vi "bigcryo_Harry-IcH - v5.vi"() -> ()   [LabVIEW 2019]
uses:
  Global 2.vi
  <vilib>/Utility/file.llb/Read From Spreadsheet File (DBL).vi
panel:
  out "Sample Temp [K] - Meas":dbl=1.55928
  out "Sample Temp - Idle [K]":dbl
  in  "LakeShore340":refnum<visa-resource-name>="COM7"
  out "dV/dI-I":cluster{dbl[], dbl[]}(graph) caption="XY Graph"
  out "I-V":cluster{dbl[], dbl[]}(graph) caption="XY Graph"
  out "Status":string="Welcome!"
  in  "Stop":bool
  in  "Keithley":refnum<visa-resource-name>="GPIB1::20::INSTR"
  in  "Delay [sec]":dbl=0.002 format="%#_6e"
  in  "Compliance [V] 2":dbl=10.0 format="%#_6f"
  in  "Delta [A]":dbl=1e-05 format="%#_6e"
  in  "Abort Conductance":bool
  in  "Step [A]":dbl=1e-05 format="%#_6e"
  in  "I-Max [A]":dbl=0.002 format="%#_6e"
  in  "Arm Conductance":bool
  in  "Measure":bool
  in  "Directory Output":string="C:\\User Data\\hlb54\\210111_42B\\JJ1\\IcH_pos_to_neg_T=4p00K_set=0p0T"
  out "B Now":string="-0.202"
  out "error out 6":errorcluster
  in  "Minicryo":bool=TRUE
  in  "Field and rate":dbl[][](array[numeric])
  in  "step":bool=TRUE
  in  "Set Rate (T/min)":dbl=0.1
  in  "Magnet VISA?":refnum<visa-resource-name>="COM6"
  out "?":refnum<visa-resource-name>="GPIB0::20::INSTR"
  out "Iteration?":i32=401
  out "Path Out":path=path "C:/User Data/Sachio/gigi.dat"
  in  "Start Field (T)":dbl=0.2 format="%#_7f"
  in  "Mag Field Step":dbl=0.002
  out "B Aim":dbl=-0.202
  in  "Stop Field":dbl=-0.2
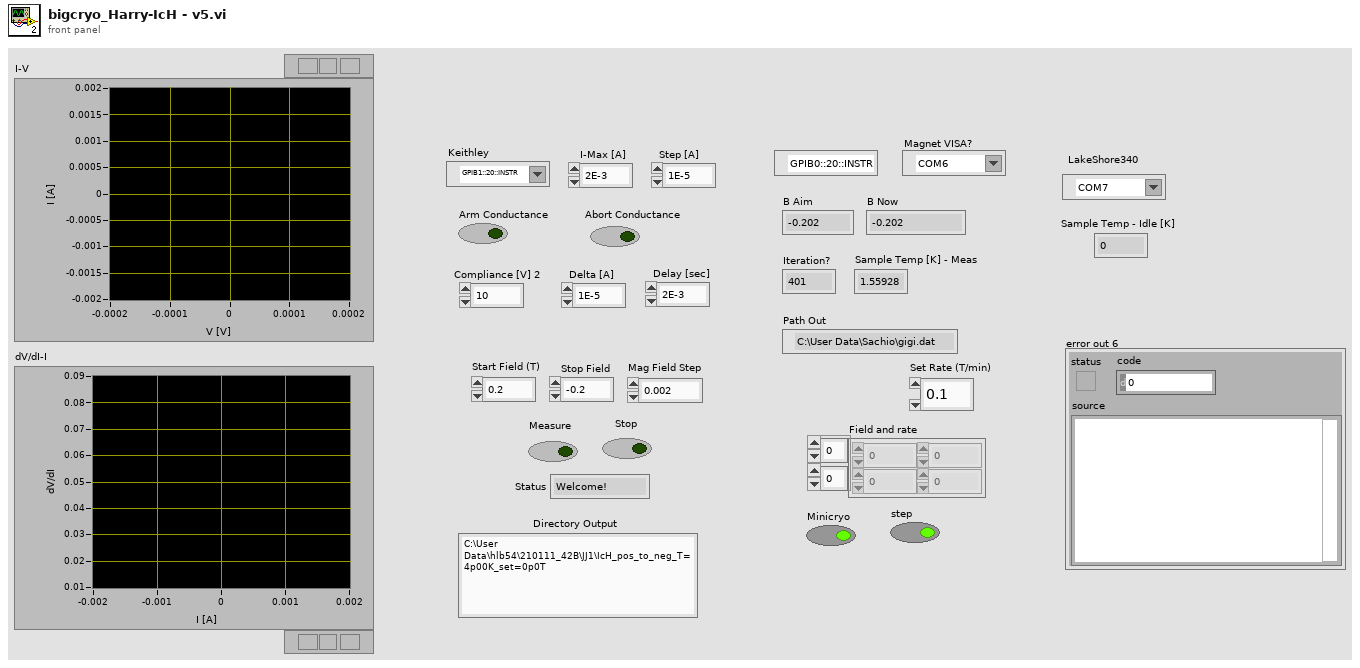
[diagram p1: front panel]
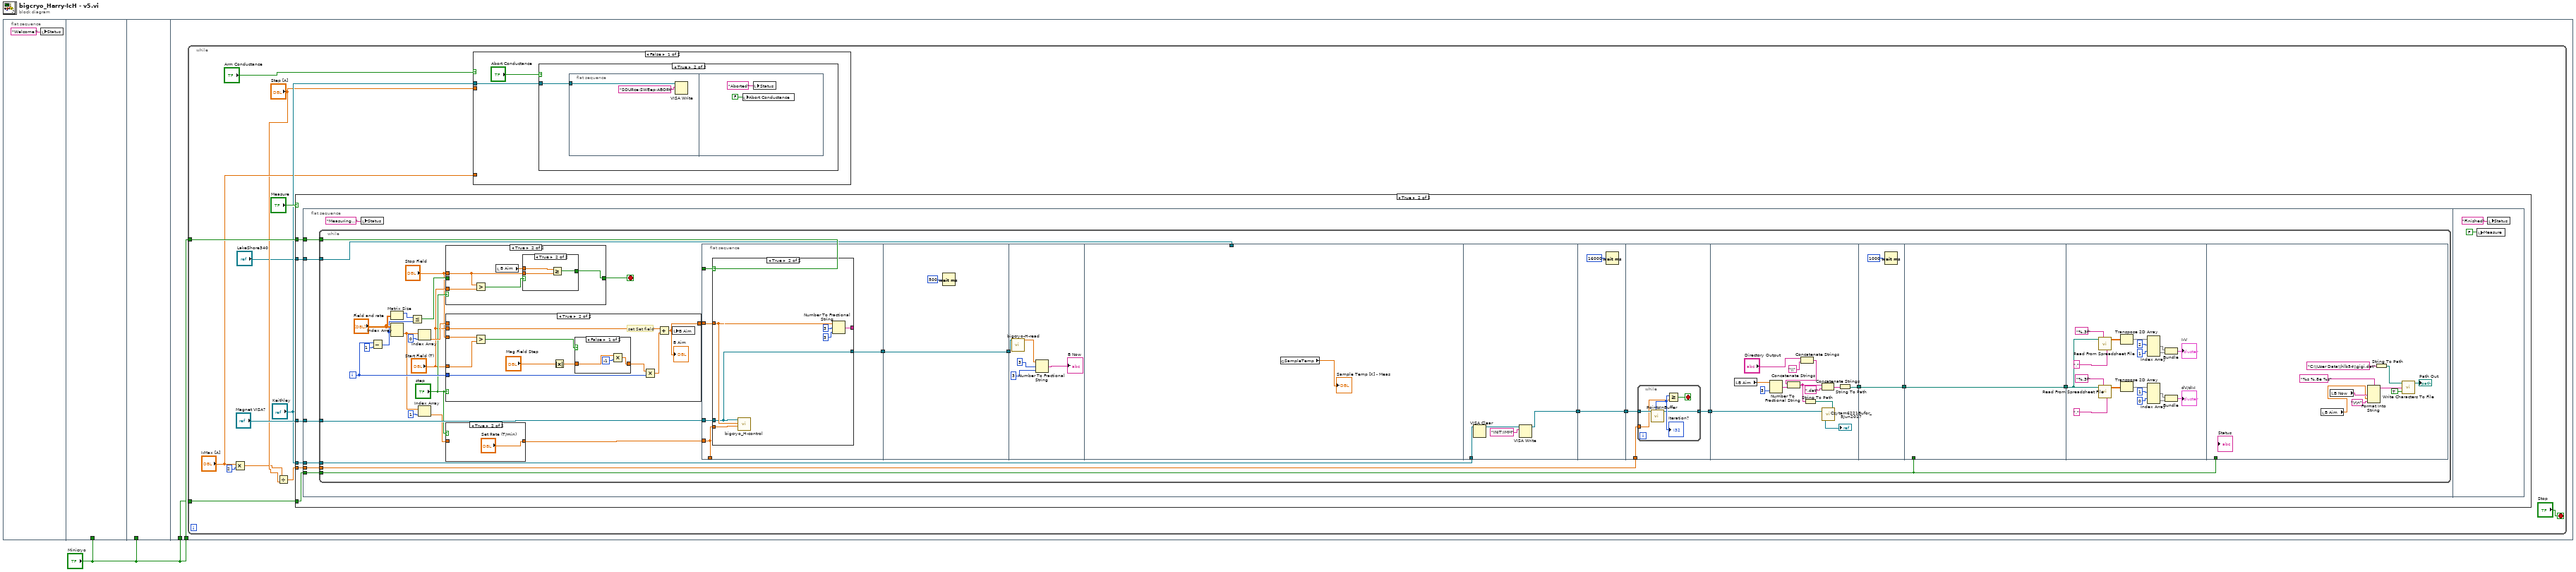
[diagram p0: block diagram]
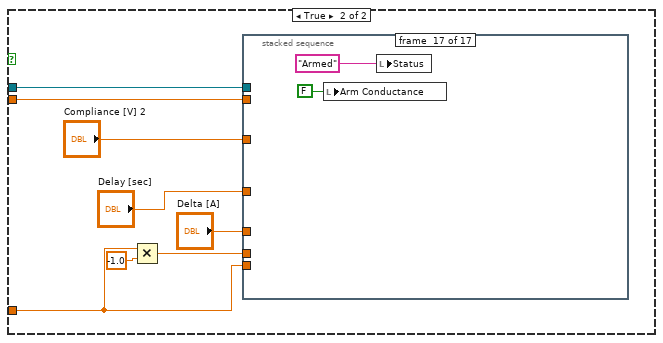
[diagram p3: hidden frame]
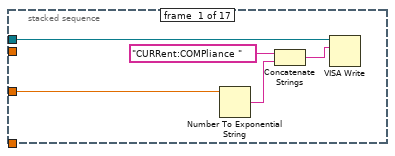
[diagram p4: hidden frame]
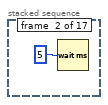
[diagram p5: hidden frame]
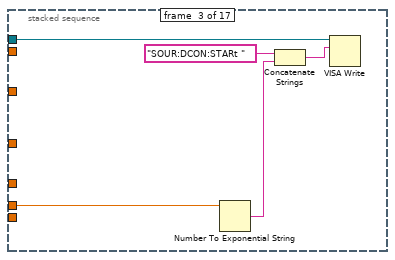
[diagram p6: hidden frame]
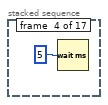
[diagram p7: hidden frame]
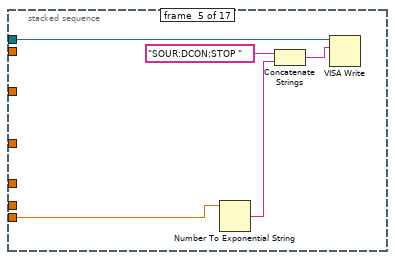
[diagram p8: hidden frame]
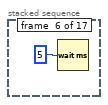
[diagram p9: hidden frame]
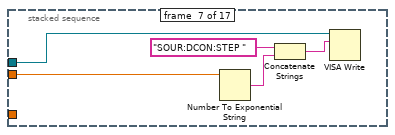
[diagram p10: hidden frame]
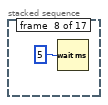
[diagram p11: hidden frame]
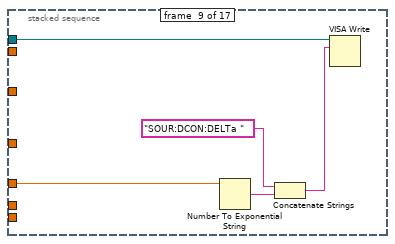
[diagram p12: hidden frame]
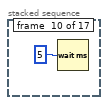
[diagram p13: hidden frame]
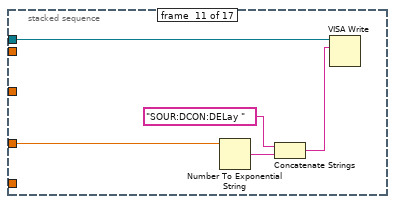
[diagram p14: hidden frame]
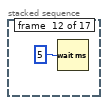
[diagram p15: hidden frame]
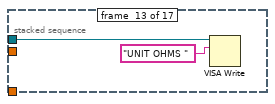
[diagram p16: hidden frame]
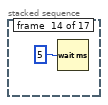
[diagram p17: hidden frame]
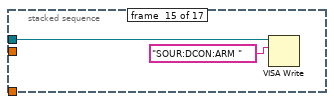
[diagram p18: hidden frame]
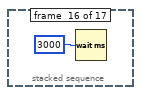
[diagram p19: hidden frame]
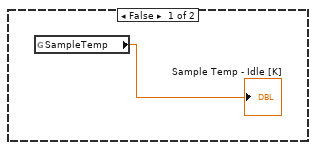
[diagram p20: hidden frame]
diagram:
  n1 = flat-sequence {
    tunnel: "Minicryo" -> [_]
    tunnel: "Minicryo" -> [_]
    tunnel: "Minicryo" -> [w4]
    tunnel: "Minicryo" -> [w3]
    frame #0 {
      n2 = local write "Status"("Welcome!") -> ()
    }
    frame #1 {
    }
    frame #2 {
    }
    frame #3 {
      n3 = while {
        tunnel: w4 -> [w16]
        tunnel: w3 -> [w15]
        stop <- "Stop" stop-if-true
        n4 = Multiply(x="I-Max [A]", y=2) -> (x*y=w6:dbl)
        n5 = Divide(x=w6, y="Step [A]") -> (x/y=w7:dbl)
        n6 = case shown="True" "Measure" {
          tunnel: "Magnet VISA?" -> [_ w83]
          tunnel: w16 -> [_ w82]
          tunnel: w15 -> [_ w81]
          tunnel: "Keithley" -> [_ w80]
          tunnel: w7 -> [_ w79]
          tunnel: "LakeShore340" -> [_ w78]
          frame False {
            n7 = global read "Global 2.vi" "SampleTemp"() -> (→"Sample Temp - Idle [K]":dbl)
          }
          frame True {
            n8 = flat-sequence {
              tunnel: w83 -> [w90]
              tunnel: w82 -> [w89]
              tunnel: w81 -> [w88]
              tunnel: w80 -> [w87]
              tunnel: w79 -> [w86]
              tunnel: w78 -> [w84]
              frame #0 {
                n9 = while {
                  tunnel: w90 -> [w117]
                  tunnel: w89 -> [w108]
                  tunnel: w88 -> [w103]
                  tunnel: w87 -> [w101]
                  tunnel: w86 -> [w100]
                  tunnel: w84 -> [w93]
                  i -> [w114]
                  stop <- w99 stop-if-true
                  n10 = Subtract(x=w114, y=1) -> (x-y=w105:i32)
                  n11 = Matrix Size(0:"Field and rate") -> (1:w106:i32)  [unwired: 1 out]
                  n12 = Index Array(array="Field and rate", index (row)=w105) -> (element=w111:dbl[])  [unwired: 1 in]
                  n13 = Less Or Equal?(x=w106, y=w105) -> (x <= y?=w104:bool)
                  n14 = Index Array(array=w111, index=0) -> (element=w110:dbl)
                  n15 = Index Array(array=w111, index=1) -> (element=w109:dbl)
                  n16 = case shown="True" "step" {
                    tunnel: [w122 w127] -> w99
                    tunnel: w104 -> [w122 _]
                    tunnel: "Stop Field" -> [_ w125]
                    tunnel: "Start Field (T)" -> [_ w124]
                    frame False {
                    }
                    frame True {
                      n17 = Greater?(x=w125, y=w124) -> (0:w123:bool)
                      n18 = local read "B Aim"() -> (w126:dbl)
                      n19 = case shown="True" w123 {
                        tunnel: [w130 w133] -> w127
                        tunnel: w126 -> [w128 w132]
                        tunnel: w125 -> [w129 w131]
                        frame False {
                          n20 = Less Or Equal?(x=w128, y=w129) -> (x <= y?=w130:bool)
                        }
                        frame True {
                          n21 = Greater Or Equal?(x=w132, y=w131) -> (x >= y?=w133:bool)
                        }
                      }
                    }
                  }
                  n22 = case shown="True" "step" {
                    tunnel: [w136 w145] -> w121
                    tunnel: w114 -> [_ w144]
                    tunnel: w110 -> [w136 _]
                    tunnel: "Start Field (T)" -> [_ w143]
                    tunnel: "Start Field (T)" -> [_ w142]
                    tunnel: "Stop Field" -> [_ w141]
                    frame False {
                    }
                    frame True {
                      # "set Set field"
                      n23 = Greater?(x=w141, y=w142) -> (0:w137:bool)
                      n24 = Absolute Value(x="Mag Field Step") -> (abs(x)=w139:dbl)
                      n25 = case shown="False" w137 {
                        tunnel: [w149 w150] -> w138
                        tunnel: w139 -> [w147 w150]
                        frame False {
                          n26 = Multiply(x=w147, y=-1) -> (x*y=w149:dbl)
                        }
                        frame True {
                        }
                      }
                      n27 = Multiply(x=w138, y=w144) -> (x*y=w146:dbl)
                      n28 = Add(x=w143, y=w146) -> (x+y=w145:dbl)
                      "B Aim" <- w145
                      n29 = local write "B Aim"(w145) -> ()
                    }
                  }
                  n30 = case shown="True" "step" {
                    tunnel: [w134 "Set Rate (T/min)"] -> w116
                    tunnel: w109 -> [w134 _]
                    frame False {
                    }
                    frame True {
                    }
                  }
                  n31 = flat-sequence {
                    tunnel: w121 -> [w155]
                    tunnel: w117 -> [w154]
                    tunnel: [w153] -> _
                    tunnel: w116 -> [w153]
                    tunnel: w108 -> [w152]
                    tunnel: [w151] -> w92
                    tunnel: w92 -> [w172]
                    tunnel: [w172] -> w91
                    tunnel: w91 -> [w174]
                    tunnel: w93 -> [_]
                    tunnel: [w181] -> w119
                    tunnel: w101 -> [w180]
                    tunnel: [w185] -> w120
                    tunnel: w119 -> [w185]
                    tunnel: w120 -> [w188]
                    tunnel: [w187] -> w118
                    tunnel: w100 -> [w186]
                    tunnel: w118 -> [w201]
                    tunnel: [w197] -> w94
                    tunnel: [w207] -> w95
                    tunnel: w94 -> [w207]
                    tunnel: w103 -> [_]
                    tunnel: [w209] -> w96
                    tunnel: w95 -> [w209]
                    tunnel: w96 -> [w210]
                    tunnel: w103 -> [_]
                    frame #0 {
                      n32 = case shown="True" w152 {
                        tunnel: w155 -> [w159 w168]
                        tunnel: w154 -> [w156 w166]
                        tunnel: w153 -> [_ w171]
                        tunnel: [w157 w167] -> _
                        tunnel: [w156 w166] -> w151
                        frame False {
                          n33 = Number To Fractional String(number=w159, width (-)=i16 3, precision (6)=i16 3) -> (F-format string=w157:string)  [unwired: 1 in]
                          n34 = Concatenate Strings("J" ("string"), w157) -> (w158:string)
                          n35 = GPIB Write(0:"25" ("address string"), 1:w158, 2:6) -> (6:→"error out 6":errorcluster)  [unwired: 2 in, 1 out]
                        }
                        frame True {
                          n36 = call "bigcryo_H-control.vi"("Rate [T/min]"=w171, "Set Field [T]"=w168, "Magnet Power supply"=w166) -> ()  [unwired: 9 in]
                          n37 = Number To Fractional String(number=w168, width (-)=i16 3, precision (6)=i16 3) -> (F-format string=w167:string)  [unwired: 1 in]
                        }
                      }
                    }
                    frame #1 {
                      n38 = Wait (ms)(milliseconds to wait=u32 500) -> ()  [unwired: 1 out]
                    }
                    frame #2 {
                      n39 = call "bigcryo-H-read.vi"("Magnet Power supply"=w174) -> ("Magnetic Field [T]"=w178:dbl)  [unwired: 9 in, 1 out]
                      n40 = Number To Fractional String(number=w178, width (-)=i16 3, precision (6)=i16 3) -> (F-format string=→"B Now":string)  [unwired: 1 in]
                    }
                    frame #3 {
                      n41 = global read "Global 2.vi" "SampleTemp"() -> (→"Sample Temp [K] - Meas":dbl)
                    }
                    frame #4 {
                      n42 = VISA Clear(VISA resource name=w180) -> (VISA resource name out=w183:refnum<visa-resource-name>)  [unwired: 1 in, 1 out]
                      n43 = VISA Write(VISA resource name=w183, write buffer="INIT:IMM") -> (VISA resource name out=w181:refnum<visa-resource-name>)  [unwired: 1 in, 2 out]
                    }
                    frame #5 {
                      n44 = Wait (ms)(milliseconds to wait=16000) -> ()  [unwired: 1 out]
                    }
                    frame #6 {
                      n45 = while {
                        tunnel: w188 -> [w191]
                        tunnel: [w190] -> w187
                        tunnel: w186 -> [w189]
                        stop <- w192 stop-if-true
                        n46 = call "PointsInBuffer.vi"("VISA resource name"=w191) -> (3:w190:refnum<visa-resource-name>, "number"=w193:i32)  [unwired: 9 in]
                        "Iteration?" <- w193
                        n47 = Greater Or Equal?(x=w193, y=w189) -> (x >= y?=w192:bool)
                      }
                    }
                    frame #7 {
                      n48 = local read "B Aim"() -> (w202:dbl)
                      n49 = Number To Fractional String(number=w202, precision (6)=i16 3) -> (F-format string=w206:string)  [unwired: 2 in]
                      n50 = Concatenate Strings("Directory Output", "\\") -> (w194:string)
                      n51 = Concatenate Strings(w194, w206) -> (w199:string)
                      n52 = String To Path(string=w199) -> (path=w205:path)
                      n53 = Concatenate Strings(w199, ".dat") -> (w198:string)
                      n54 = call "Czytam6221Bufor_5Jun2017.vi"("file path (dialog if empty)"=w205, 3:w201) -> (2:→"?":refnum<visa-resource-name>)  [unwired: 1 in]
                      n55 = String To Path(string=w198) -> (path=w197:path)
                    }
                    frame #8 {
                      n56 = Wait (ms)(milliseconds to wait=u32 1000) -> ()  [unwired: 1 out]
                    }
                    frame #9 {
                    }
                    frame #10 {
                      n57 = call-poly <vilib>:"Read From Spreadsheet File.vi"("delimiter (\\t)"="," ("delimiter (\\t)"), "format (%.3f)"="%.3f", "file path (dialog if empty)"=w210) -> ("all rows"=w223:dbl[][])  [unwired: 4 in, 4 out]
                      n58 = call-poly <vilib>:"Read From Spreadsheet File.vi"("delimiter (\\t)"="," ("delimiter (\\t)"), "format (%.3f)"="%.3f", "file path (dialog if empty)"=w210) -> ("all rows"=w214:dbl[][])  [unwired: 4 in, 4 out]
                      n59 = Transpose 2D Array(2D array=w223) -> (transposed array=w222:dbl[][])
                      n60 = Transpose 2D Array(2D array=w214) -> (transposed array=w213:dbl[][])
                      n61 = Index Array(array=w222, index (row) #1=2 ("index (row)"), index (row) #2=1 ("index (row)")) -> (element #1=w225:dbl[], element #2=w224:dbl[])  [unwired: 2 in]
                      n62 = Index Array(array=w213, index (row) #1=1 ("index (row)"), index (row) #2=0 ("index (row)")) -> (element #1=w216:dbl[], element #2=w215:dbl[])  [unwired: 2 in]
                      n63 = Bundle(w225, w224) -> (→"I-V":cluster{dbl[], dbl[]})  [unwired: 1 in]
                      n64 = Bundle(w216, w215) -> (→"dV/dI-I":cluster{dbl[], dbl[]})  [unwired: 1 in]
                    }
                    frame #11 {
                      n65 = local read "B Aim"() -> (w229:dbl)
                      n66 = local read "B Now"() -> (w232:string)
                      n67 = Format Into String(format string="%s %.8e %s", w232, w229, "\r\n") -> (resulting string=w235:string)  [unwired: 2 in, 1 out]
                      n68 = String To Path(string="C:\\User Data\\hlb54\\gigi.dat") -> (path=w230:path)
                      n69 = call "Write Characters To File.vi"("append to file? (new file:F)"=TRUE, "character string"=w235, "file path (dialog if empty)"=w230) -> ("new file path (Not A Path if cancelled)"=→"Path Out":path)  [unwired: 1 in, 1 out]
                    }
                  }
                }
                n70 = local write "Status"("Measuring...") -> ()
              }
              frame #1 {
                n71 = local write "Measure"(FALSE) -> ()
                n72 = local write "Status"("Finished") -> ()
              }
            }
          }
        }
        n73 = case shown="False" "Arm Conductance" {
          tunnel: "Keithley" -> [w18 w28]
          tunnel: "Step [A]" -> [_ w27]
          tunnel: "I-Max [A]" -> [_ w25]
          frame False {
            n74 = case shown="True" "Abort Conductance" {
              tunnel: w18 -> [_ w20]
              frame False {
              }
              frame True {
                n75 = flat-sequence {
                  tunnel: w20 -> [w21]
                  frame #0 {
                    n76 = VISA Write(VISA resource name=w21, write buffer="SOURce:SWEep:ABORt") -> ()  [unwired: 1 in, 3 out]
                  }
                  frame #1 {
                    n77 = local write "Abort Conductance"(FALSE) -> ()
                    n78 = local write "Status"("Aborted") -> ()
                  }
                }
              }
            }
          }
          frame True {
            n79 = Multiply(x=w25, y=-1.0) -> (x*y=w26:dbl)
            n80 = stacked-sequence {
              tunnel: w26 -> [_ _ w41 _ _ _ _ _ _ _ _ _ _ _ _ _ _]
              tunnel: "Delay [sec]" -> [_ _ _ _ _ _ _ _ _ _ w64 _ _ _ _ _ _]
              tunnel: "Compliance [V] 2" -> [w34 _ _ _ _ _ _ _ _ _ _ _ _ _ _ _ _]
              tunnel: "Delta [A]" -> [_ _ _ _ _ _ _ _ w58 _ _ _ _ _ _ _ _]
              tunnel: w28 -> [w33 _ w39 _ w46 _ w52 _ w57 _ w63 _ w69 _ w72 _ _]
              tunnel: w27 -> [_ _ _ _ _ _ w51 _ _ _ _ _ _ _ _ _ _]
              tunnel: w25 -> [_ _ _ _ w45 _ _ _ _ _ _ _ _ _ _ _ _]
              frame #0 {
                n81 = Number To Exponential String(number=w34) -> (E-format string=w36:string)  [unwired: 3 in]
                n82 = Concatenate Strings("CURRent:COMPliance ", w36) -> (w35:string)
                n83 = VISA Write(VISA resource name=w33, write buffer=w35) -> ()  [unwired: 1 in, 3 out]
              }
              frame #1 {
                n84 = Wait (ms)(milliseconds to wait=5) -> ()  [unwired: 1 out]
              }
              frame #2 {
                n85 = Number To Exponential String(number=w41) -> (E-format string=w42:string)  [unwired: 3 in]
                n86 = Concatenate Strings("SOUR:DCON:STARt ", w42) -> (w40:string)
                n87 = VISA Write(VISA resource name=w39, write buffer=w40) -> ()  [unwired: 1 in, 3 out]
              }
              frame #3 {
                n88 = Wait (ms)(milliseconds to wait=5) -> ()  [unwired: 1 out]
              }
              frame #4 {
                n89 = Number To Exponential String(number=w45) -> (E-format string=w48:string)  [unwired: 3 in]
                n90 = Concatenate Strings("SOUR:DCON:STOP ", w48) -> (w47:string)
                n91 = VISA Write(VISA resource name=w46, write buffer=w47) -> ()  [unwired: 1 in, 3 out]
              }
              frame #5 {
                n92 = Wait (ms)(milliseconds to wait=5) -> ()  [unwired: 1 out]
              }
              frame #6 {
                n93 = Number To Exponential String(number=w51) -> (E-format string=w54:string)  [unwired: 3 in]
                n94 = Concatenate Strings("SOUR:DCON:STEP ", w54) -> (w53:string)
                n95 = VISA Write(VISA resource name=w52, write buffer=w53) -> ()  [unwired: 1 in, 3 out]
              }
              frame #7 {
                n96 = Wait (ms)(milliseconds to wait=5) -> ()  [unwired: 1 out]
              }
              frame #8 {
                n97 = Number To Exponential String(number=w58) -> (E-format string=w60:string)  [unwired: 3 in]
                n98 = Concatenate Strings("SOUR:DCON:DELTa ", w60) -> (w59:string)
                n99 = VISA Write(VISA resource name=w57, write buffer=w59) -> ()  [unwired: 1 in, 3 out]
              }
              frame #9 {
                n100 = Wait (ms)(milliseconds to wait=5) -> ()  [unwired: 1 out]
              }
              frame #10 {
                n101 = Number To Exponential String(number=w64) -> (E-format string=w66:string)  [unwired: 3 in]
                n102 = Concatenate Strings("SOUR:DCON:DELay ", w66) -> (w65:string)
                n103 = VISA Write(VISA resource name=w63, write buffer=w65) -> ()  [unwired: 1 in, 3 out]
              }
              frame #11 {
                n104 = Wait (ms)(milliseconds to wait=5) -> ()  [unwired: 1 out]
              }
              frame #12 {
                n105 = VISA Write(VISA resource name=w69, write buffer="UNIT OHMS ") -> ()  [unwired: 1 in, 3 out]
              }
              frame #13 {
                n106 = Wait (ms)(milliseconds to wait=5) -> ()  [unwired: 1 out]
              }
              frame #14 {
                n107 = VISA Write(VISA resource name=w72, write buffer="SOUR:DCON:ARM ") -> ()  [unwired: 1 in, 3 out]
              }
              frame #15 {
                n108 = Wait (ms)(milliseconds to wait=3000) -> ()  [unwired: 1 out]
              }
              frame #16 {
                n109 = local write "Arm Conductance"(FALSE) -> ()
                n110 = local write "Status"("Armed") -> ()
              }
            }
          }
        }
      }
    }
  }
